vi "2700多功能.vi"() -> ()   [LabVIEW 2019]
uses:
  <instrlib>/Keithley 27XX/Public/Configure/Measurement Specific/Configure FRTD.vi
  <instrlib>/Keithley 27XX/Public/Data/Read Multiple Direct.vi
  <instrlib>/Keithley 27XX/Keithley 27XX.lvlib
panel:
  out "Measurement Data":dbl[](array[numeric])
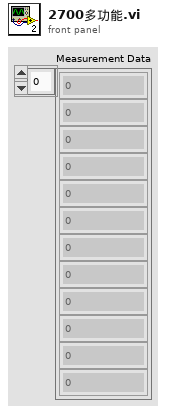
[diagram p1: front panel]
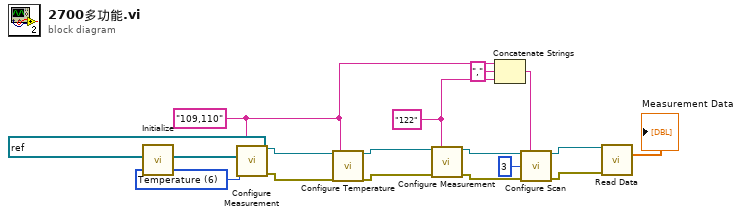
[diagram p0: block diagram]
diagram:
  w8 = "122" ("Scan List (Empty)")
  w9 = "109,110" ("Scan List (Empty)")
  w16 = u16 6 items=["DC Voltage", "AC Voltage", "DC Current", "AC Current", "Resistance", "Four-Wire Resistance", "Temperature", "Frequency", "Period", "Continuity"] ("Function (0: DC Voltage)")
  n1 = call <instrlib>:"Initialize.vi"("VISA resource name"=refnum<visa-resource-name> "USB0::0x05E6::0x6510::04434284::INSTR") -> ("VISA resource name out"=w17:refnum<visa-resource-name>)  [unwired: 13 in, 1 out]
  n2 = call <instrlib>:"Configure Measurement.vi"("VISA resource name"=w17, "Scan List (Empty)"=w9, "Function (0: DC Voltage)"=w16) -> ("VISA resource name out"=w15:refnum<visa-resource-name>, "error out"=w14:errorcluster)  [unwired: 11 in]
  n3 = call-poly <instrlib>:"Configure Temperature.vi"("VISA resource name"=w15, "error in (no error)"=w14, "Scan List (Empty)"=w9) -> ("VISA resource name out"=w13:refnum<visa-resource-name>, "error out"=w12:errorcluster)  [unwired: 15 in]
  n4 = call <instrlib>:"Configure Measurement.vi"("VISA resource name"=w13, "Scan List (Empty)"=w8, "error in (no error)"=w12) -> ("VISA resource name out"=w11:refnum<visa-resource-name>, "error out"=w10:errorcluster)  [unwired: 11 in]
  n5 = Concatenate Strings(w9, "," ("字符串"), w8) -> (w6:string)
  n6 = call <instrlib>:"Configure Scan.vi"("VISA resource name"=w11, "Channel List (101:110)"=w6, "Sample Count (100)"=3, "error in (no error)"=w10) -> ("VISA resource name out"=w4:refnum<visa-resource-name>, "error out"=w3:errorcluster)  [unwired: 10 in]
  n7 = call-poly <instrlib>:"Read Data.vi"("VISA resource name"=w4, "error in (no error)"=w3) -> ("Measurement Data"=→"Measurement Data":dbl[])  [unwired: 8 in, 5 out]
